vi "Previous Settings Dialog.vi"(8 "error in (no error)":errorcluster, 11 "Settings in":T1={"Hardware Configuration"={"VISA resource name"="", "DAQ Type"=enum."Simulated", "Channel 1"={"Acquiring"=FALSE, "Enabled"=FALSE, "Terminal configuration"=32767, "Range"=0}, "Channel 2"={"Acquiring"=FALSE, "Enabled"=FALSE, "Terminal configuration"=0, "Range"=0}, "Timing"={"Sample Rate"=0, "Actual Sample Rate"=0, "Samples per Iteration"=0, "Sample Clock Source"=0, "Time Units"=0}, "PS Parameters"={"PS handle"=0, "PS Max_adc"=32767, "PS Enabled Array"=[], "PS Device Info"={"Driver Version"="", "USB Version"="", "Hardware"="", "Variant"="", "Batch and Serial"="", "Cal Date"="", "Kernel Version"="", "Digital HW Version"="", "Analogue HW Version"="", "Firmware 1"="", "Firmware 2"="", "MSO"=FALSE, "Number of Channels"=0}, "Channel 1 Buffer"=refnum, "Channel 2 Buffer"=refnum}, "Trigger"={"Direction"=0, "Threshold [V]"=0.0, "Enabled"=FALSE, "Trigger Source"=0}, "Keithley Parameters"={"Previous End / Current Start"=0}}, "Logging Configuration"={"Log File Base Path"=path "", "TDMS File Reference"=refnum, "Enabled"=FALSE}} {"Hardware Configuration"."Trigger"."Trigger Source" items=["Channel 1"=0, "Channel 2"=1, "Ext."=4]; "Hardware Configuration"."Trigger"."Direction" items=["Channel 1", "Channel 2", "External"]; "Hardware Configuration"."Timing"."Time Units" items=["Seconds"]; "Hardware Configuration"."Timing"."Sample Clock Source" items=["Internal", "External"]; "Hardware Configuration"."Channel 2"."Terminal configuration" items=["Referenced Single Ended", "Differential"]; "Hardware Configuration"."Channel 1"."Terminal configuration" items=["Referenced Single Ended", "Differential"]}) -> (0 "error out":errorcluster, 1 "Cancelled?":bool, 2 "UI Refresh Needed?":bool, 3 "Settings out":T1={"Hardware Configuration"={"VISA resource name"="", "DAQ Type"=enum."Simulated", "Channel 1"={"Acquiring"=FALSE, "Enabled"=FALSE, "Terminal configuration"=32767, "Range"=0}, "Channel 2"={"Acquiring"=FALSE, "Enabled"=FALSE, "Terminal configuration"=0, "Range"=0}, "Timing"={"Sample Rate"=0, "Actual Sample Rate"=0, "Samples per Iteration"=0, "Sample Clock Source"=0, "Time Units"=0}, "PS Parameters"={"PS handle"=0, "PS Max_adc"=32767, "PS Enabled Array"=[], "PS Device Info"={"Driver Version"="", "USB Version"="", "Hardware"="", "Variant"="", "Batch and Serial"="", "Cal Date"="", "Kernel Version"="", "Digital HW Version"="", "Analogue HW Version"="", "Firmware 1"="", "Firmware 2"="", "MSO"=FALSE, "Number of Channels"=0}, "Channel 1 Buffer"=refnum, "Channel 2 Buffer"=refnum}, "Trigger"={"Direction"=0, "Threshold [V]"=0.0, "Enabled"=FALSE, "Trigger Source"=0}, "Keithley Parameters"={"Previous End / Current Start"=0}}, "Logging Configuration"={"Log File Base Path"=path "", "TDMS File Reference"=refnum, "Enabled"=FALSE}} {"Hardware Configuration"."Trigger"."Trigger Source" items=["Channel 1"=0, "Channel 2"=1, "Ext."=4]; "Hardware Configuration"."Trigger"."Direction" items=["Channel 1", "Channel 2", "External"]; "Hardware Configuration"."Timing"."Time Units" items=["Seconds"]; "Hardware Configuration"."Timing"."Sample Clock Source" items=["Internal", "External"]; "Hardware Configuration"."Channel 2"."Terminal configuration" items=["Referenced Single Ended", "Differential"]; "Hardware Configuration"."Channel 1"."Terminal configuration" items=["Referenced Single Ended", "Differential"]})   [LabVIEW 2016]
doc: "Dialog for selecting user specified settings."
uses:
  Settings.ctl
  Acquisition/Hardware Configuration.ctl
  Acquisition/Signal Type.ctl
  Logging/Logging Configuration.ctl
  <vilib>/Utility/xml.llb/Write to XML File(string).vi
  Settings.lvlib
  Acquisition/Acquisition.lvlib
  Logging/Logging.lvlib
panel:
  in  "Time Unit":u16(ring) items=["ns"=2, "us"=3, "ms"=4, "s"=5]
  in  "Tab Control":enum32{"Disabled", "Analog", "Digital"}(tab)
  in  "Direction":u16(ring) items=["Rising"=3, "Falling"=4]
  in  "Threshold [V]":dbl
  in  "Trigger Source":u16(ring) items=["Channel 1"=0, "Channel 2"=1, "External"=4]
  in  "On/Off":bool=TRUE
  in  "Range [V]":u16(ring) items=["0.01", "0.02", "0.05", "0.1", "0.2", "0.5", "1", "2", "5", "10", "20", "50", "100"]
  in  "Range [V]":u16(ring) items=["0.01", "0.02", "0.05", "0.1", "0.2", "0.5", "1", "2", "5", "10", "20", "50", "100"]
  out "Samples per Iteration":dbl
  out "Actual Samping Time":dbl
  in  "Sampling Time":u32=1
  in  "Sample Clock Source":u16(ring) items=["Internal", "External"]
  out "Acquiring 2":bool
  out "Acquiring":bool
  in  "Terminal configuration":u16(ring) items=["Referenced Single Ended", "Differential"]
  in  "Physical connection":u16(ring) items=["Disabled", "Channel 1", "Channel 2"]
  in  "Terminal configuration":u16(ring) items=["Referenced Single Ended", "Differential"]
  in  "Physical connection":u16(ring) items=["Disabled", "Channel 1", "Channel 2"]
  in  "VISA resource name":refnum<visa-resource-name>
  in  "Log File Path":path
  in  "DAQ Type":u16(ring) items=["Simulated", "Tektronics DPO2k/3k/4k", "PicoScope 2000a Series", "Keithley DMM7510", "PicoScope 5000a Series"]
  in  "Cancel Button":bool
  in  "OK Button":bool
  # "Non visible portion of dialog (needed for connector pane)."
  # "Timing Settings"
  # "Channel Settings (Signal 1)"
  # "Trigger Settings"
  # "Channel Settings (Signal 2)"
  # "Logging"
  # "To configure and use a start trigger you must select\nthe specific tab. Not all hardware supports triggering.\nRefer to your device documentation for more info"
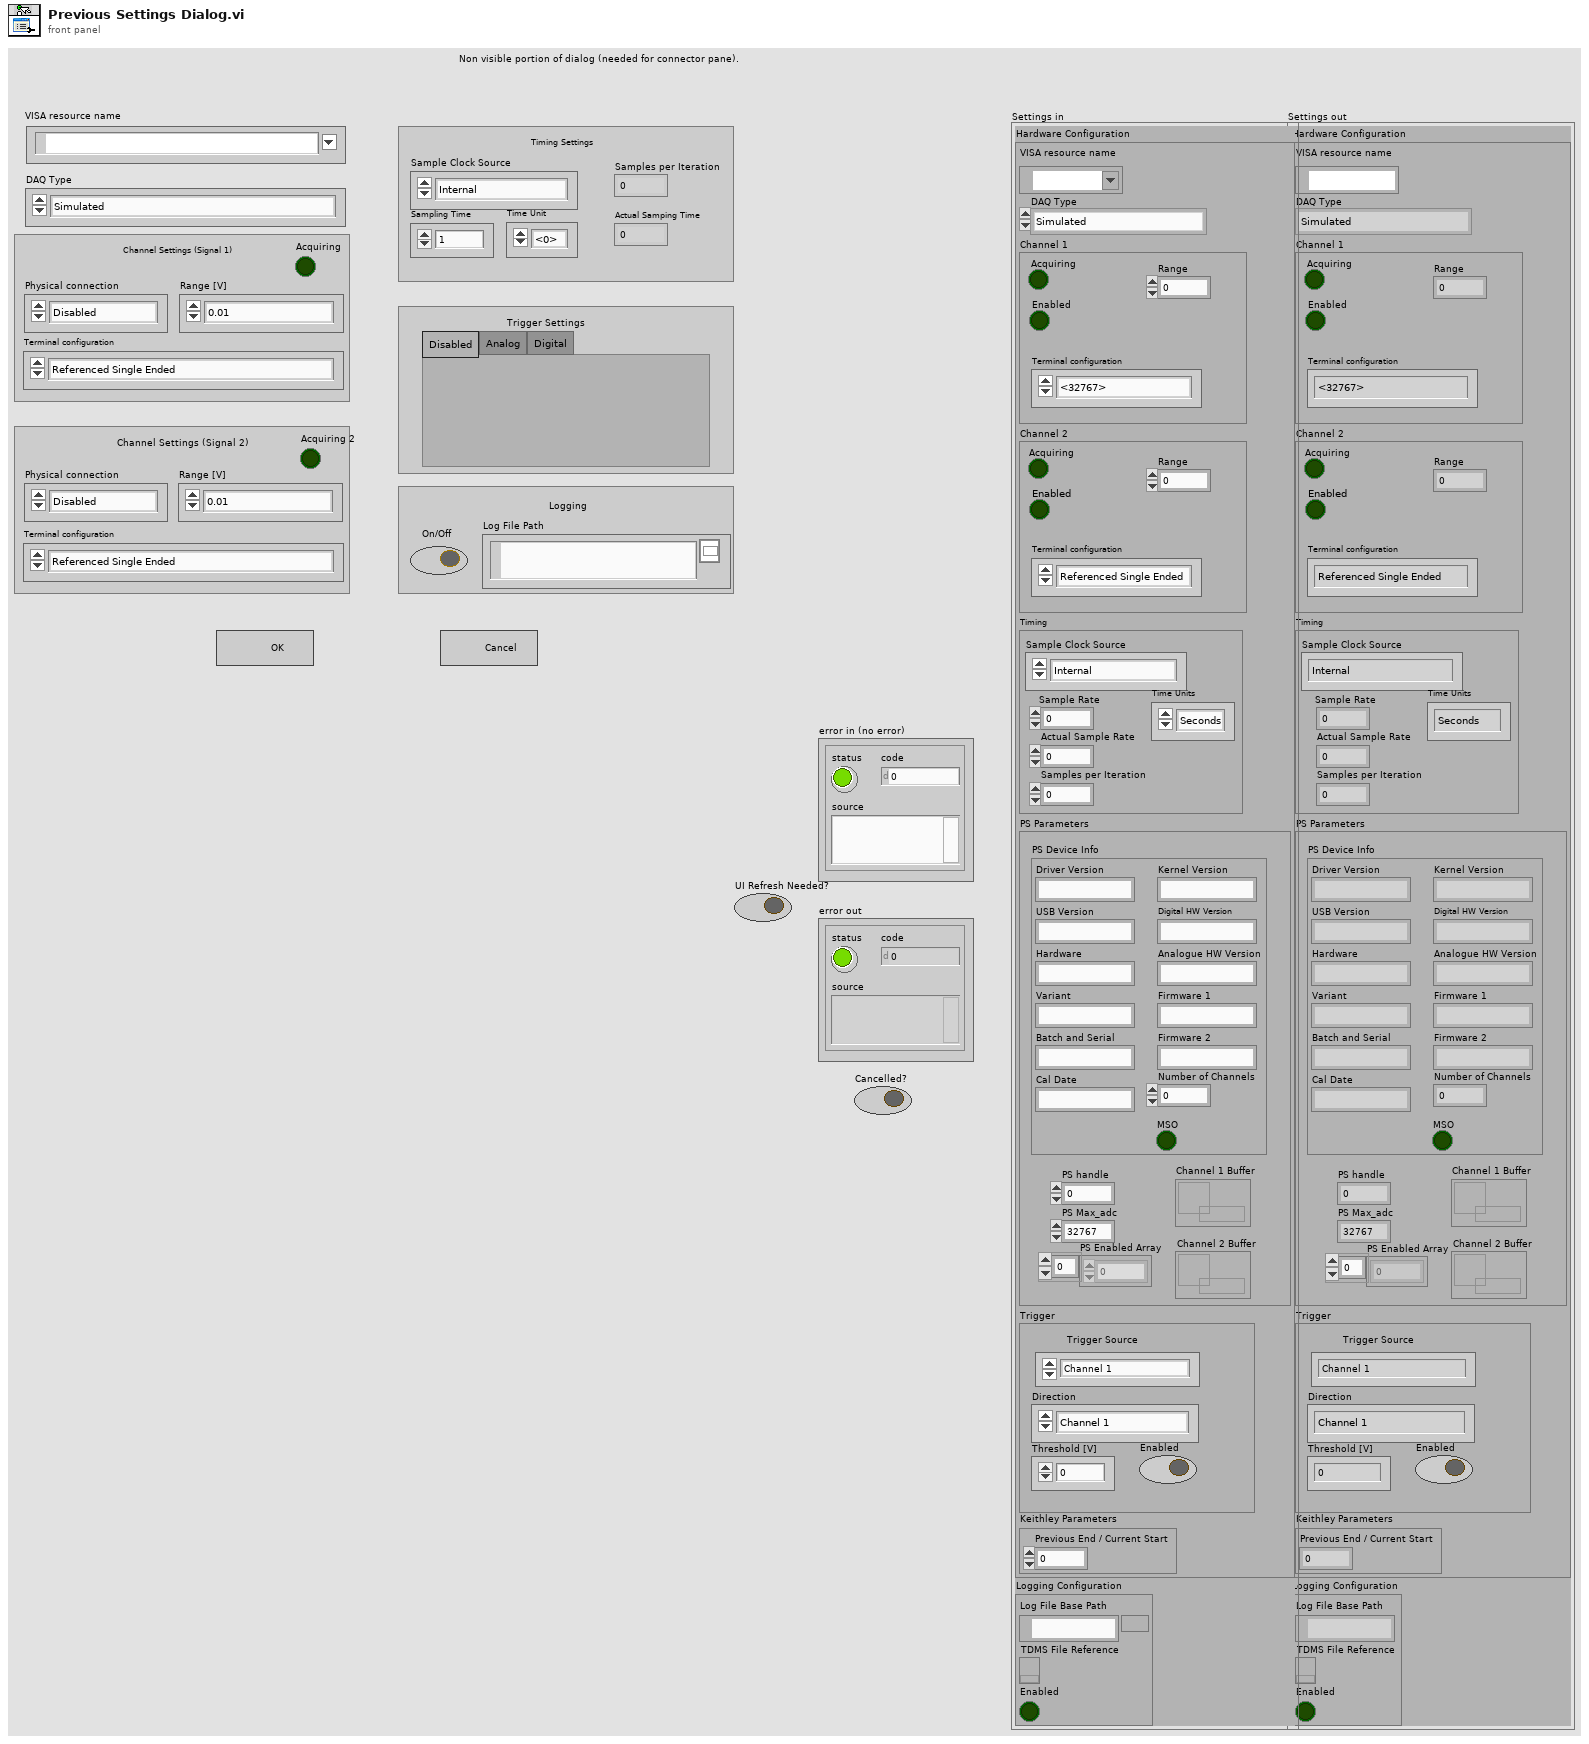
[diagram p1: front panel]
types:
  T1 = typedef "Settings.lvlib/Settings.ctl" = cluster{"Hardware Configuration":T2, "Logging Configuration":T4}
  T2 = typedef "Acquisition.lvlib/Hardware Configuration.ctl" = cluster{"VISA resource name":refnum<visa-resource-name>, "DAQ Type":T3, "Channel 1":cluster{"Acquiring":bool, "Enabled":bool, "Terminal configuration":u16, "Range":u16}, "Channel 2":cluster{"Acquiring":bool, "Enabled":bool, "Terminal configuration":u16, "Range":u16}, "Timing":cluster{"Sample Rate":u32, "Actual Sample Rate":u32, "Samples per Iteration":u32, "Sample Clock Source":u16, "Time Units":u32}, "PS Parameters":cluster{"PS handle":i16, "PS Max_adc":i16, "PS Enabled Array":i16[], "PS Device Info":cluster{"Driver Version":string, "USB Version":string, "Hardware":string, "Variant":string, "Batch and Serial":string, "Cal Date":string, "Kernel Version":string, "Digital HW Version":string, "Analogue HW Version":string, "Firmware 1":string, "Firmware 2":string, "MSO":bool, "Number of Channels":i16}, "Channel 1 Buffer":refnum<data-value>, "Channel 2 Buffer":refnum<data-value>}, "Trigger":cluster{"Direction":u16, "Threshold [V]":dbl, "Enabled":bool, "Trigger Source":u16}, "Keithley Parameters":cluster{"Previous End / Current Start":i32}}
  T3 = typedef "Acquisition.lvlib/Signal Type.ctl" = enum16{"Simulated", "Tektronics DPO2k/3k/4k", "PicoScope 2000a Series", "Keithley DMM7510", "PicoScope 5000a Series"}
  T4 = typedef "Logging.lvlib/Logging Configuration.ctl" = cluster{"Log File Base Path":path, "TDMS File Reference":refnum<k34>, "Enabled":bool}
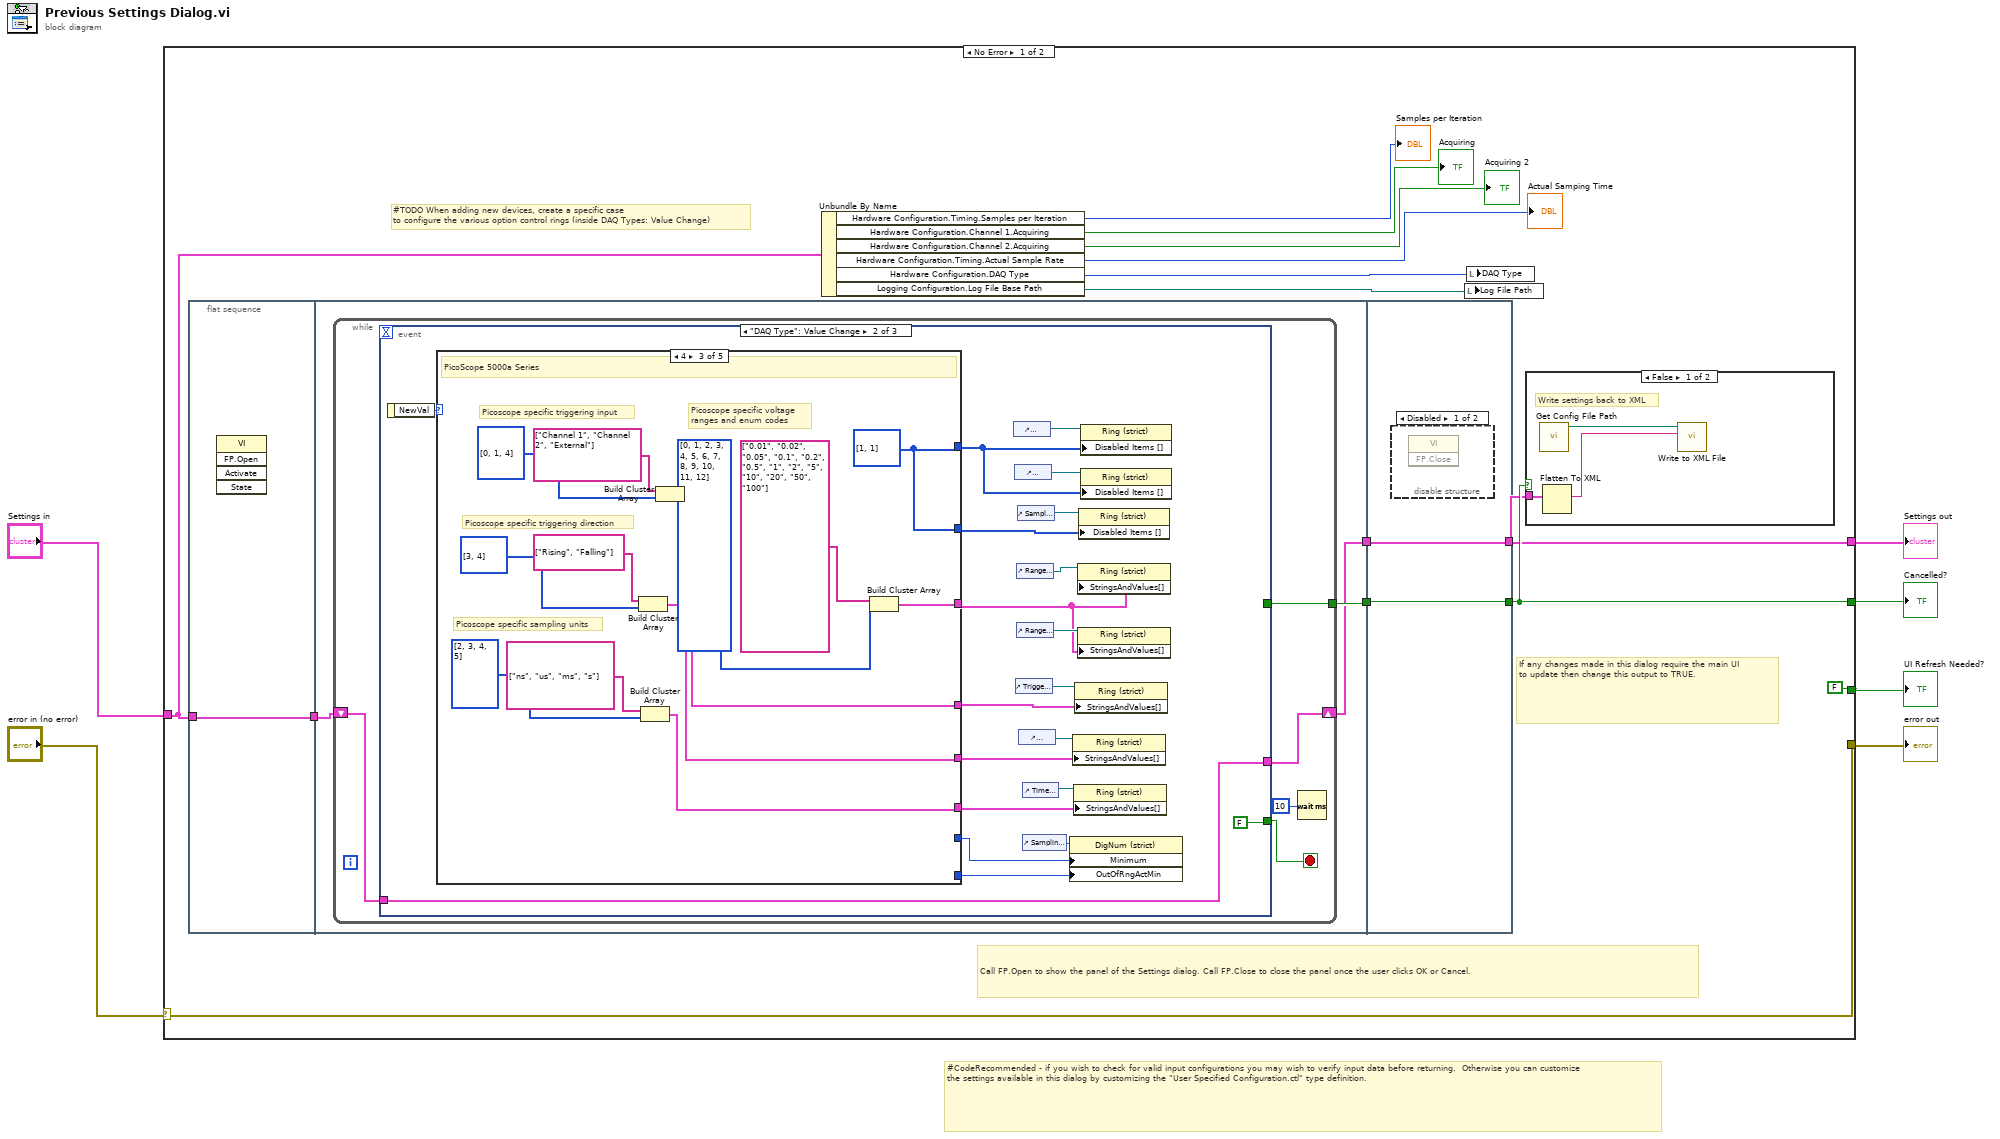
[diagram p0: block diagram]
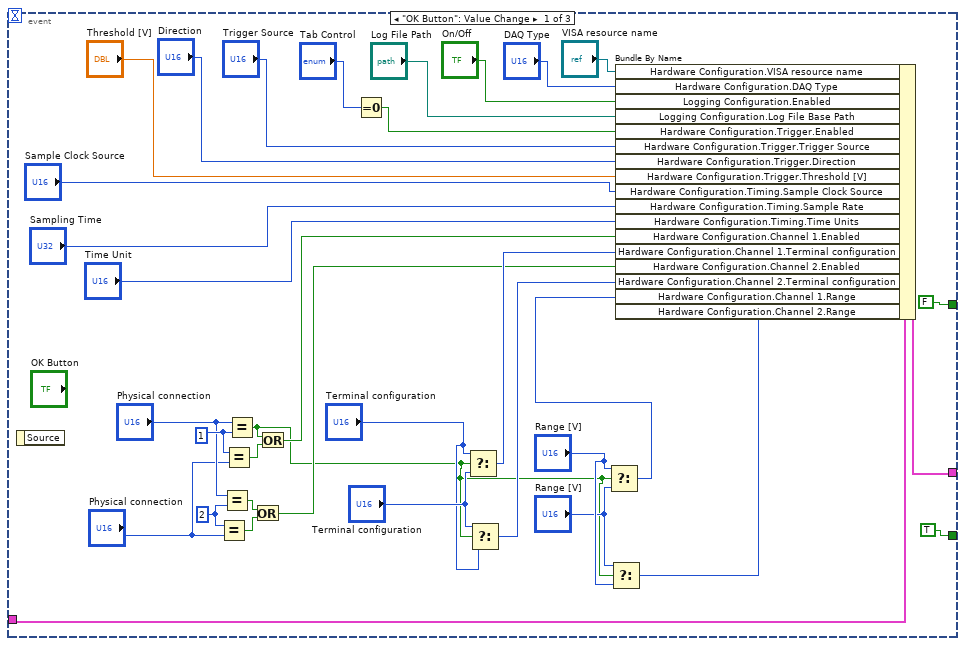
[diagram p2: hidden frame]
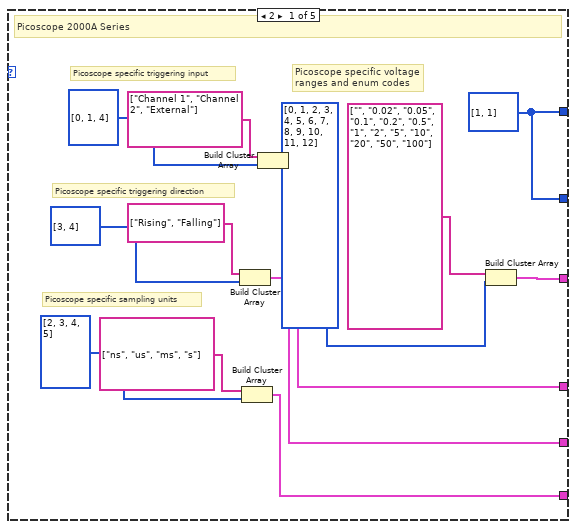
[diagram p3: hidden frame]
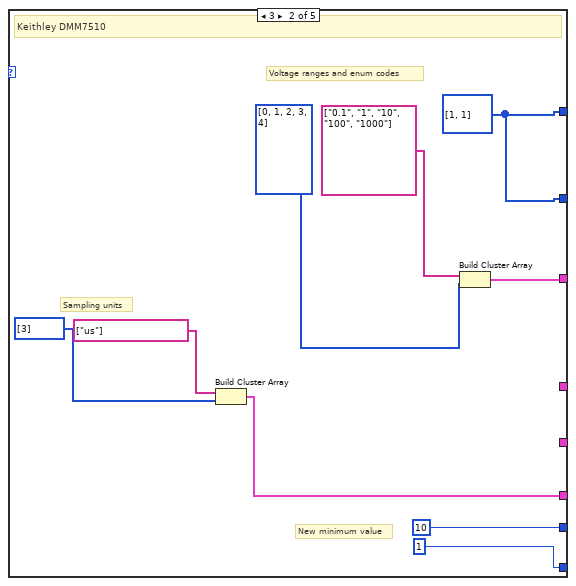
[diagram p4: hidden frame]
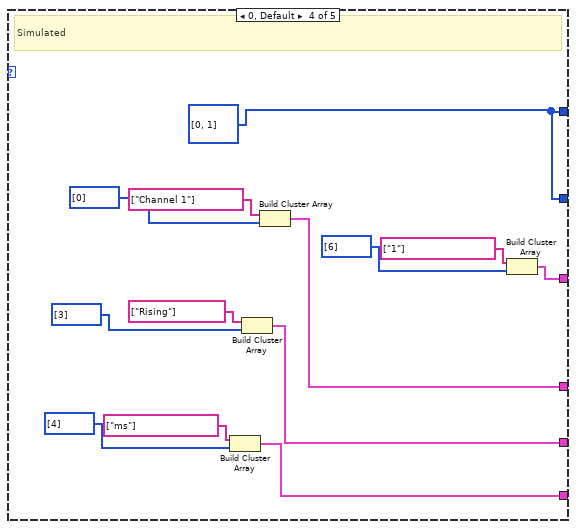
[diagram p5: hidden frame]
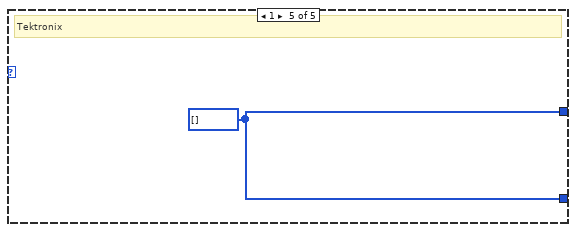
[diagram p6: hidden frame]
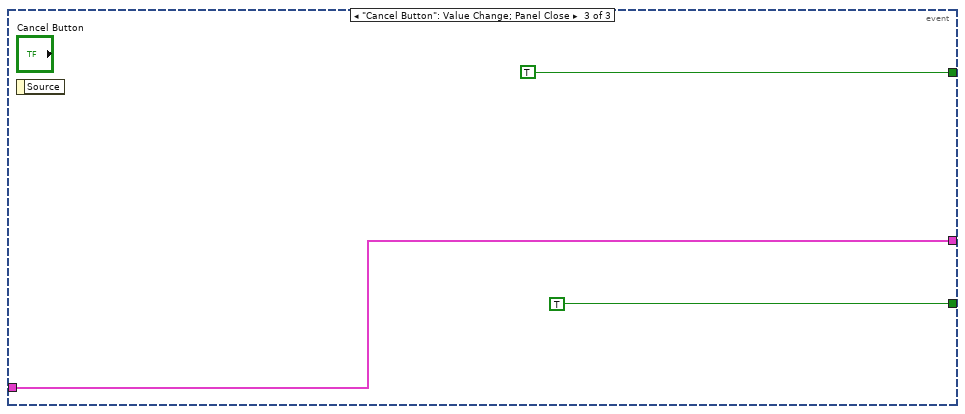
[diagram p7: hidden frame]
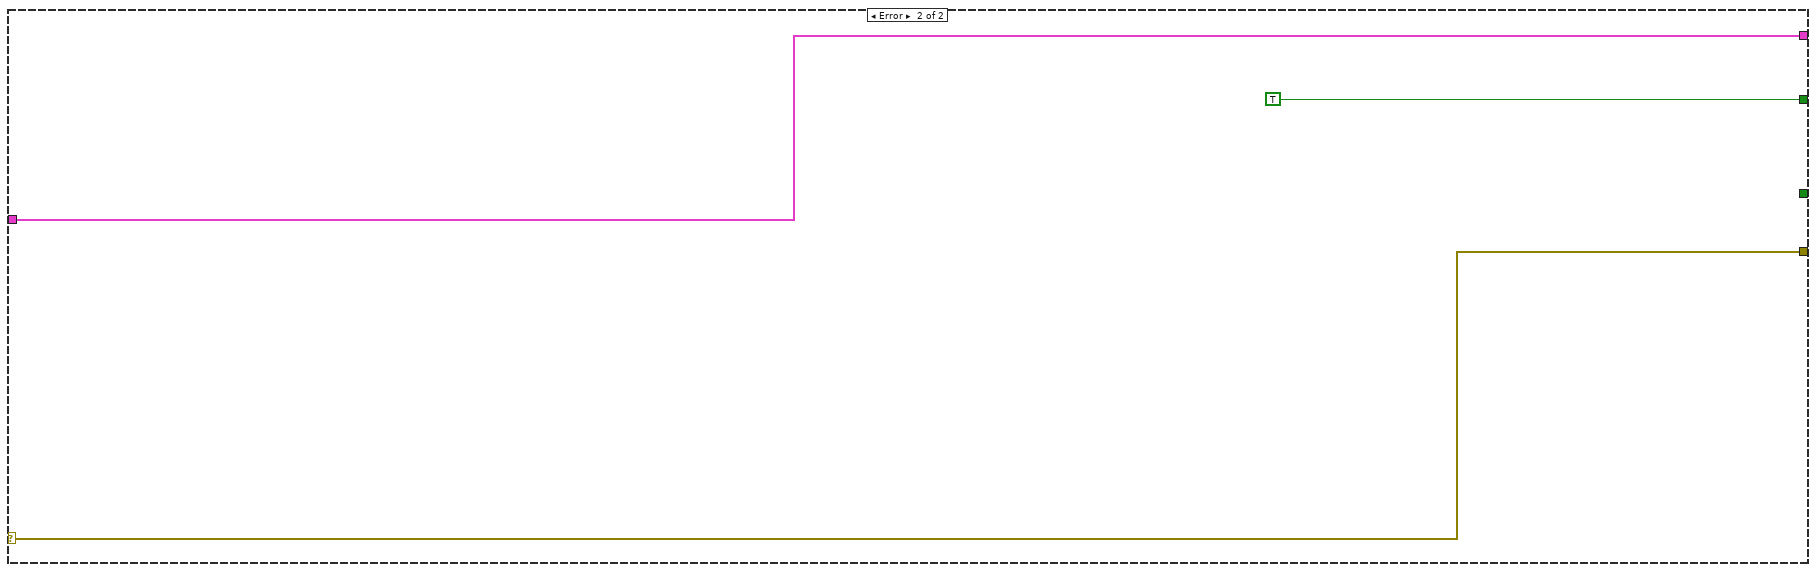
[diagram p10: hidden frame]
diagram:
  # "#CodeRecommended - if you wish to check for valid input configurations you may wish to verify input data before returning.  Otherwise you can customize the settings available in this dialog by customizing the \"User Specified Configuration.ctl\" type definition."
  n1 = case shown="No Error" "error in (no error)" {
    selector: "error in (no error)" -> [w20 w143]
    tunnel: [w20 w143] -> w5
    tunnel: "Settings in" -> [w16 w142]
    tunnel: [w17 w142] -> w3
    tunnel: [FALSE ("UI Refresh Needed?") _] -> w2
    tunnel: [w18 TRUE ("UI Refresh Needed?")] -> w1
    frame No Error {
      # "#TODO When adding new devices, create a specific case\nto configure the various option control rings (inside DAQ Types: Value Change)"
      # "Call FP.Open to show the panel of the Settings dialog. Call FP.Close to close the panel once the user clicks OK or Cancel."
      # "If any changes made in this dialog require the main UI to update then change this output to TRUE."
      n2 = flat-sequence {
        tunnel: w16 -> [w21]
        tunnel: [w21] -> w13
        tunnel: w13 -> [w22]
        tunnel: [w24] -> w12
        tunnel: [w23] -> w11
        tunnel: [w136] -> w17
        tunnel: [w137] -> w18
        tunnel: w12 -> [w137]
        tunnel: w11 -> [w136]
        frame #0 {
          n3 = invoke class="VI" method="FP.Open"() -> ()  [unwired: 5 in, 5 out]
        }
        frame #1 {
          n4 = while {
            tunnel: [w29] -> w24
            shift-right: [w28] -> w23
            shift-left: w22 -> [w27]
            stop <- w26 stop-if-true
            n5 = event shown="[1] \"DAQ Type\": Value Change" {
              selector: _ -> [_ _ _]
              dyn-events: _ -> [_ _ _]
              timeout: _ -> [_ _ _]
              tunnel: [w61 w83 w135] -> w28
              tunnel: w27 -> [w62 w83 w135]
              tunnel: [FALSE ("UI Refresh Needed?") _ TRUE ("UI Refresh Needed?")] -> w29
              tunnel: [TRUE FALSE TRUE] -> w26
              event "OK Button": Value Change {
                w54 = u16 2 ("x")
                w56 = u16 1 ("x")
                n6 = event-data() -> ()  [unwired: 1 in, 1 out]
                n7 = Equal?(x=w54, y="Physical connection") -> (x = y?=w53:bool)
                n8 = Equal?(x="Physical connection", y=w54) -> (x = y?=w43:bool)
                n9 = Equal?(x=w56, y="Physical connection") -> (x = y?=w55:bool)
                n10 = Equal?(x="Physical connection", y=w56) -> (x = y?=w34:bool)
                n11 = Or(x=w43, y=w53) -> (x .or. y?=w47:bool)
                n12 = Or(x=w34, y=w55) -> (x .or. y?=w40:bool)
                n13 = Equal To 0?(x="Tab Control") -> (x = 0?=w38:bool)
                n14 = Select(t="Terminal configuration", s=w34, f="Terminal configuration") -> (s? t:f=w48:u16)
                n15 = Select(t="Terminal configuration", s=w34, f="Terminal configuration") -> (s? t:f=w46:u16)
                n16 = Select(t="Range [V]", s=w34, f="Range [V]") -> (s? t:f=w42:u16)
                n17 = Select(t="Range [V]", s=w34, f="Range [V]") -> (s? t:f=w33:u16)
                n18 = Bundle By Name(cluster=w62, "Hardware Configuration.VISA resource name"="VISA resource name", "Hardware Configuration.DAQ Type"="DAQ Type", "Logging Configuration.Enabled"="On/Off", "Logging Configuration.Log File Base Path"="Log File Path", "Hardware Configuration.Trigger.Enabled"=w38, "Hardware Configuration.Trigger.Trigger Source"="Trigger Source", "Hardware Configuration.Trigger.Direction"="Direction", "Hardware Configuration.Trigger.Threshold [V]"="Threshold [V]", "Hardware Configuration.Timing.Sample Clock Source"="Sample Clock Source", "Hardware Configuration.Timing.Sample Rate"="Sampling Time", "Hardware Configuration.Timing.Time Units"="Time Unit", "Hardware Configuration.Channel 1.Enabled"=w40, "Hardware Configuration.Channel 1.Terminal configuration"=w48, "Hardware Configuration.Channel 2.Enabled"=w47, "Hardware Configuration.Channel 2.Terminal configuration"=w46, "Hardware Configuration.Channel 1.Range"=w42, "Hardware Configuration.Channel 2.Range"=w33) -> (w61:T1)
              }
              event "DAQ Type": Value Change {
                n19 = event-data() -> ("NewVal"=w82:u16)  [unwired: 1 in]
                n20 = case shown="4" w82 {
                  tunnel: [w96 w100 w109 w127 w132] -> w77
                  tunnel: [w96 w100 w109 w127 w132] -> w76
                  tunnel: [w95 w99 w110 w128 _] -> w73
                  tunnel: [w90 _ w108 w129 _] -> w71
                  tunnel: [w87 _ w107 w130 _] -> w69
                  tunnel: [w84 w101 w106 w131 _] -> w68
                  tunnel: [_ 10 _ _ _] -> w65
                  tunnel: [_ u8 1 ("Response to Value Outside Limits:Minimum") _ _ _] -> w64
                  frame 2 {
                    w96 = i32[] [1, 1] ("Disabled Items []")
                    # "Picoscope specific sampling units"
                    # "Picoscope specific triggering direction"
                    # "Picoscope specific triggering input"
                    # "Picoscope specific voltage \nranges and enum codes"
                    # "Picoscope 2000A Series"
                    n21 = Build Cluster Array(string[] ["Rising", "Falling"], i32[] [3, 4]) -> (w87:cluster{string, i32}[])
                    n22 = Build Cluster Array(string[] ["ns", "us", "ms", "s"], i32[] [2, 3, 4, 5]) -> (w84:cluster{string, i32}[])
                    n23 = Build Cluster Array(string[] ["Channel 1", "Channel 2", "External"], i32[] [0, 1, 4]) -> (w90:cluster{string, i32}[])
                    n24 = Build Cluster Array(string[] ["", "0.02", "0.05", "0.1", "0.2", "0.5", "1", "2", "5", "10", "20", "50", "100"], u16[] [0, 1, 2, 3, 4, 5, 6, 7, 8, 9, 10, 11, 12]) -> (w95:cluster{string, u16}[])
                  }
                  frame 3 {
                    w100 = i32[] [1, 1] ("Disabled Items []")
                    # "New minimum value"
                    # "Sampling units"
                    # "Voltage ranges and enum codes"
                    # "Keithley DMM7510"
                    n25 = Build Cluster Array(string[] ["us"], i32[] [3]) -> (w101:cluster{string, i32}[])
                    n26 = Build Cluster Array(string[] ["0.1", "1", "10", "100", "1000"], u16[] [0, 1, 2, 3, 4]) -> (w99:cluster{string, u16}[])
                  }
                  frame 4 {
                    w109 = i32[] [1, 1] ("Disabled Items []")
                    # "Picoscope specific sampling units"
                    # "Picoscope specific triggering direction"
                    # "Picoscope specific triggering input"
                    # "Picoscope specific voltage \nranges and enum codes"
                    # "PicoScope 5000a Series"
                    n27 = Build Cluster Array(string[] ["Rising", "Falling"], i32[] [3, 4]) -> (w107:cluster{string, i32}[])
                    n28 = Build Cluster Array(string[] ["ns", "us", "ms", "s"], i32[] [2, 3, 4, 5]) -> (w106:cluster{string, i32}[])
                    n29 = Build Cluster Array(string[] ["Channel 1", "Channel 2", "External"], i32[] [0, 1, 4]) -> (w108:cluster{string, i32}[])
                    n30 = Build Cluster Array(string[] ["0.01", "0.02", "0.05", "0.1", "0.2", "0.5", "1", "2", "5", "10", "20", "50", "100"], u16[] [0, 1, 2, 3, 4, 5, 6, 7, 8, 9, 10, 11, 12]) -> (w110:cluster{string, u16}[])
                  }
                  frame 0, Default {
                    w127 = i32[] [0, 1] ("Disabled Items []")
                    # "Simulated"
                    n31 = Build Cluster Array(string[] ["ms"], i32[] [4]) -> (w131:cluster{string, i32}[])
                    n32 = Build Cluster Array(string[] ["Rising"], i32[] [3]) -> (w130:cluster{string, i32}[])
                    n33 = Build Cluster Array(string[] ["Channel 1"], i32[] [0]) -> (w129:cluster{string, i32}[])
                    n34 = Build Cluster Array(string[] ["1"], i32[] [6]) -> (w128:cluster{string, i32}[])
                  }
                  frame 1 {
                    w132 = u16[] []
                    # "Tektronix"
                  }
                }
                n35 = control-ref of="Terminal configuration"() -> (w80:refnum<vi>)
                n36 = control-ref of="Terminal configuration"() -> (w79:refnum<vi>)
                n37 = control-ref of="Trigger Source"() -> (w72:refnum<vi>)
                n38 = control-ref of="Range [V]"() -> (w75:refnum<vi>)
                n39 = control-ref of="Range [V]"() -> (w74:refnum<vi>)
                n40 = control-ref of="Sample Clock Source"() -> (w78:refnum<vi>)
                n41 = control-ref of="Direction"() -> (w70:refnum<vi>)
                n42 = control-ref of="Time Unit"() -> (w67:refnum<vi>)
                n43 = control-ref of="Sampling Time"() -> (w66:refnum<vi>)
                n44 = property class="DigNum (strict)"(reference=w66, "Minimum"=w65, "OutOfRngActMin"=w64) -> ()  [unwired: 1 in, 2 out]
                n45 = property class="Ring (strict)"(reference=w70, "StringsAndValues[]"=w69) -> ()  [unwired: 1 in, 2 out]
                n46 = property class="Ring (strict)"(reference=w67, "StringsAndValues[]"=w68) -> ()  [unwired: 1 in, 2 out]
                n47 = property class="Ring (strict)"(reference=w72, "StringsAndValues[]"=w71) -> ()  [unwired: 1 in, 2 out]
                n48 = property class="Ring (strict)"(reference=w75, "StringsAndValues[]"=w73) -> ()  [unwired: 1 in, 2 out]
                n49 = property class="Ring (strict)"(reference=w74, "StringsAndValues[]"=w73) -> ()  [unwired: 1 in, 2 out]
                n50 = property class="Ring (strict)"(reference=w78, "Disabled Items []"=w76) -> ()  [unwired: 1 in, 2 out]
                n51 = property class="Ring (strict)"(reference=w80, "Disabled Items []"=w77) -> ()  [unwired: 1 in, 2 out]
                n52 = property class="Ring (strict)"(reference=w79, "Disabled Items []"=w77) -> ()  [unwired: 1 in, 2 out]
              }
              event "Cancel Button": Value Change; Panel Close {
                n53 = event-data() -> ()  [unwired: 1 in, 1 out]
              }
            }
            n54 = Wait (ms)(milliseconds to wait=u32 10) -> ()  [unwired: 1 out]
          }
        }
        frame #2 {
          n55 = disable-structure shown="Disabled" {
            frame Disabled {
              n56 = invoke class="VI" method="FP.Close"() -> ()  [unwired: 3 in, 3 out]
            }
            frame Enabled {
            }
          }
        }
      }
      n57 = Unbundle By Name(w16) -> ("Hardware Configuration.Timing.Samples per Iteration"=→"Samples per Iteration":u32, "Hardware Configuration.Channel 1.Acquiring"=→"Acquiring":bool, "Hardware Configuration.Channel 2.Acquiring"=→"Acquiring 2":bool, "Hardware Configuration.Timing.Actual Sample Rate"=→"Actual Samping Time":u32, "Hardware Configuration.DAQ Type"=w15:T3, "Logging Configuration.Log File Base Path"=w14:path)
      n58 = local write "Log File Path"(w14) -> ()
      n59 = local write "DAQ Type"(w15) -> ()
      n60 = case shown="False" w18 {
        tunnel: w17 -> [w139 _]
        frame False {
          # "Write settings back to XML"
          n61 = call "Get Config File Path.vi"() -> ("XML File Path"=w140:path)  [unwired: 10 in, 1 out]
          n62 = Flatten To XML(anything=w139) -> (xml string=w138:string)
          n63 = call-poly <vilib>:"Write to XML File.vi"("XML Input"=w138, "XML File Path"=w140) -> ()  [unwired: 7 in, 3 out]
        }
        frame True {
        }
      }
    }
    frame Error {
    }
  }
  "UI Refresh Needed?" <- w2
  "error out" <- w5
  "Settings out" <- w3
  "Cancelled?" <- w1
